vi "FPGA Settings.vi"(6 "Action":T2, 8 "error in (no error)":errorcluster, 10 "FPGA Settings":T1={"Bitfile path"=path "", "RIO Device Address"="RIO0"}, 11 "Item Ref":T3 format="%.0x") -> (0 "error out":errorcluster, 2 "FPGA Settings":T1, 3 "Item Ref out":T3=18446744073709551615 format="%.0x")   [LabVIEW 2016, in "FPGA RM Shared API.lvlib"]
uses:
  FPGA RM Shared API.lvlib
  Types/FPGA Settings.ctl
  <vilib>/NI Veristand/Custom Device API/Custom Device Item Ref.ctl
  Types/FG Action.ctl
  <vilib>/NI Veristand/Custom Device API/Set Item Property (String).vi
  <vilib>/NI Veristand/Custom Device API/Set Item Property (Path).vi
  <vilib>/NI Veristand/Custom Device API/Get Item Property (String).vi
  <vilib>/NI Veristand/Custom Device API/Get Item Property (Path).vi
  <vilib>/NI VeriStand/Custom Device API/Custom Device API.lvlib
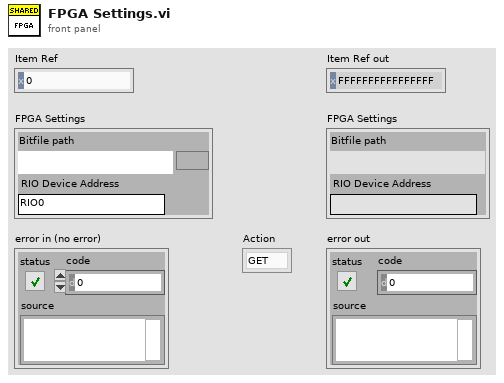
[diagram p1: front panel]
types:
  T1 = typedef "FPGA RM Shared API.lvlib/FPGA Settings.ctl" = cluster{"Bitfile path":path, "RIO Device Address":string}
  T2 = typedef "FPGA RM Shared API.lvlib/FG Action.ctl" = enum8{"GET", "SET"}
  T3 = typedef "Custom Device API.lvlib/Custom Device Item Ref.ctl" = u64
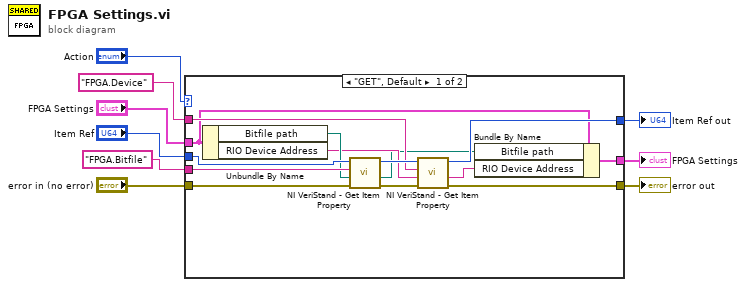
[diagram p0: block diagram]
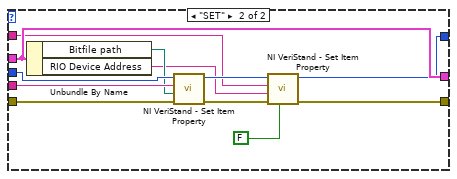
[diagram p2: hidden frame]
diagram:
  n1 = case shown="\"GET\", Default" "Action" {
    tunnel: "error in (no error)" -> [w23 w35]
    tunnel: "Item Ref" -> [w22 w34]
    tunnel: "FPGA Settings" -> [w13 w32]
    tunnel: [w17 w25] -> w9
    tunnel: [w19 w24] -> w5
    tunnel: [w12 w32] -> w3
    tunnel: "FPGA.Bitfile" ("FPGA.Bitfile") -> [w21 w33]
    tunnel: "FPGA.Device" ("FPGA.Device") -> [w14 w26]
    frame "GET", Default {
      n2 = Unbundle By Name(w13) -> ("Bitfile path"=w16:path, "RIO Device Address"=w15:string)
      n3 = call-poly <vilib>:"NI VeriStand - Get Item Property.vi"("error in (no error)"=w23, "Default Value"=w16, "Property Name"=w21, "Item Ref in"=w22) -> ("error out"=w18:errorcluster, "Value"=w11:path, "Item Ref out"=w20:T3)  [unwired: 4 in, 1 out]
      n4 = call-poly <vilib>:"NI VeriStand - Get Item Property.vi"("error in (no error)"=w18, "Default Value"=w15, "Property Name"=w14, "Item Ref in"=w20) -> ("error out"=w17:errorcluster, "Value"=w10:string, "Item Ref out"=w19:T3)  [unwired: 4 in, 1 out]
      n5 = Bundle By Name(cluster=w13, "Bitfile path"=w11, "RIO Device Address"=w10) -> (w12:T1)
    }
    frame "SET" {
      n6 = Unbundle By Name(w32) -> ("Bitfile path"=w31:path, "RIO Device Address"=w27:string)
      n7 = call-poly <vilib>:"NI VeriStand - Set Item Property.vi"("error in (no error)"=w35, "Value"=w31, "Property Name"=w33, "Item Ref in"=w34) -> ("error out"=w30:errorcluster, "Item Ref out"=w29:T3)  [unwired: 5 in, 1 out]
      n8 = call-poly <vilib>:"NI VeriStand - Set Item Property.vi"("Binary String (T)"=FALSE, "error in (no error)"=w30, "Value"=w27, "Property Name"=w26, "Item Ref in"=w29) -> ("error out"=w25:errorcluster, "Item Ref out"=w24:T3)  [unwired: 4 in, 1 out]
    }
  }
  "error out" <- w9
  "Item Ref out" <- w5
  "FPGA Settings" <- w3
